vi "Avantes - AVS_UseHighResADC.vi"(8 "error in (no error)":errorcluster, 10 "a_Enable":u8, 11 "AVS Settings In":T1) -> (0 "error out":errorcluster, 3 "AVS Settings Out":T1)   [LabVIEW 2014, in "AvaSpec.lvlib" / "Avantes Spectrometer Functions.lvlib"]
uses:
  Avantes Spectrometer Functions.lvlib
  AVS settings.ctl
  AvaSpec.lvlib
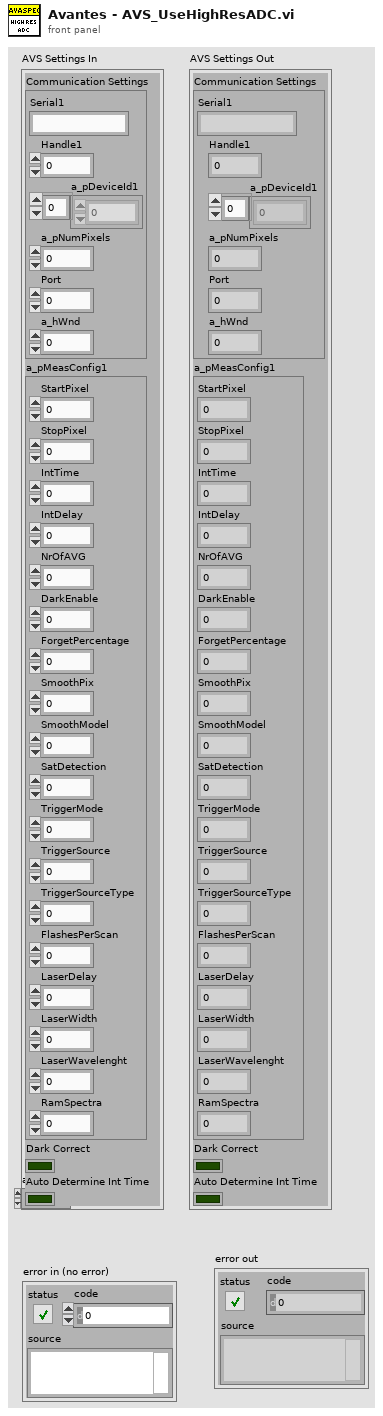
[diagram p1: front panel]
types:
  T1 = typedef "AvaSpec.lvlib/AVS settings.ctl" = cluster{"Communication Settings":cluster{"Serial1":string, "Handle1":i32, "a_pDeviceId1":u8[], "a_pNumPixels":u16, "Port":i32, "a_hWnd":i32}, "a_pMeasConfig1":cluster{"StartPixel":u16, "StopPixel":u16, "IntTime":sgl, "IntDelay":u32, "NrOfAVG":u32, "DarkEnable":u8, "ForgetPercentage":u8, "SmoothPix":u16, "SmoothModel":u8, "SatDetection":u8, "TriggerMode":u8, "TriggerSource":u8, "TriggerSourceType":u8, "FlashesPerScan":u16, "LaserDelay":u32, "LaserWidth":u32, "LaserWavelenght":sgl, "RamSpectra":u16}, "Dark Correct":bool, "Auto Determine Int Time":bool}
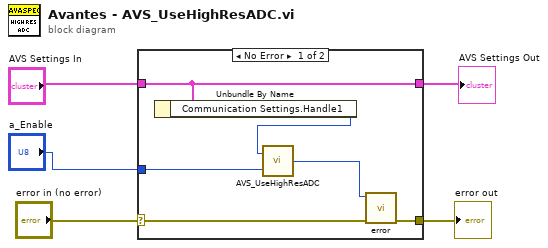
[diagram p0: block diagram]
diagram:
  n1 = case shown="No Error" "error in (no error)" {
    selector: "error in (no error)" -> [w7 w13]
    tunnel: [w11 w12] -> w1
    tunnel: "AVS Settings In" -> [w11 w12]
    tunnel: [w8 w13] -> w4
    tunnel: "a_Enable" -> [w9 _]
    frame No Error {
      n2 = Unbundle By Name(w11) -> ("Communication Settings.Handle1"=w10:i32)
      n3 = call "AVS_UseHighResADC.vi"("a_Enable"=w9, "a_hDevice"=w10) -> ("Output Value"=w6:i32)
      n4 = call "error.vi"("error in (no error)"=w7, "Output Value"=w6) -> ("error out"=w8:errorcluster)  [unwired: 9 in]
    }
    frame Error {
    }
  }
  "error out" <- w4
  "AVS Settings Out" <- w1
